vi "Merge Limelight Data.vi"   [LabVIEW 2025]
uses:
  <vilib>/Rock Robotics/Network Tables/NT Read Numeric Array.vi
  <vilib>/Rock Robotics/Network Tables/NT Read Number.vi
  Framework/Robot Global Data.vi
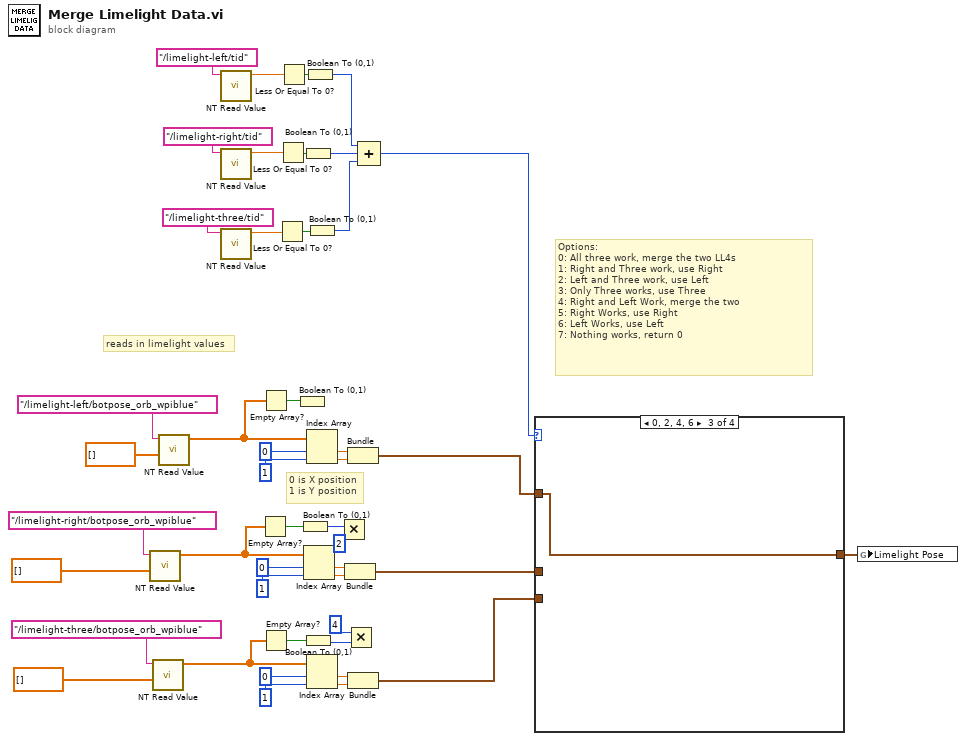
[diagram p0: block diagram]
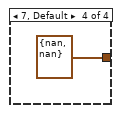
[diagram p4: hidden frame]
diagram:
  # "Options:\n0: All three work, merge the two LL4s \n1: Right and Three work, use Right\n2: Left and Three work, use Left\n3: Only Three works, use Three\n4: Right and Left Work, merge the two\n5: Right Works, use Right\n6: Left Works, use Left\n7: Nothing works, return 0"
  # "reads in limelight values"
  # "0 is X position\n1 is Y position"
  n1 = call-poly <vilib>:"NT Read Value.vi"("default value"=dbl[] [], "name"="/limelight-right/botpose_orb_wpiblue") -> ("value"=w26:dbl[])  [unwired: 7 in, 2 out]
  n2 = call-poly <vilib>:"NT Read Value.vi"("default value"=dbl[] [], "name"="/limelight-three/botpose_orb_wpiblue") -> ("value"=w25:dbl[])  [unwired: 7 in, 2 out]
  n3 = call-poly <vilib>:"NT Read Value.vi"("default value"=dbl[] [], "name"="/limelight-left/botpose_orb_wpiblue") -> ("value"=w27:dbl[])  [unwired: 7 in, 2 out]
  n4 = call-poly <vilib>:"NT Read Value.vi"("name"="/limelight-left/tid") -> ("value"=w10:dbl)  [unwired: 8 in, 2 out]
  n5 = call-poly <vilib>:"NT Read Value.vi"("name"="/limelight-right/tid") -> ("value"=w9:dbl)  [unwired: 8 in, 2 out]
  n6 = call-poly <vilib>:"NT Read Value.vi"("name"="/limelight-three/tid") -> ("value"=w8:dbl)  [unwired: 8 in, 2 out]
  n7 = Empty Array?(array=w26) -> (empty?=w23:bool)
  n8 = Empty Array?(array=w27) -> (empty?=w22:bool)
  n9 = Empty Array?(array=w25) -> (empty?=w24:bool)
  n10 = Less Or Equal To 0?(x=w8) -> (x <= 0?=w7:bool)
  n11 = Less Or Equal To 0?(x=w9) -> (x <= 0?=w6:bool)
  n12 = Less Or Equal To 0?(x=w10) -> (x <= 0?=w5:bool)
  n13 = Boolean To (0,1)(Boolean=w22) -> ()  [unwired: 1 out]
  n14 = Boolean To (0,1)(Boolean=w23) -> (0, 1=w19:i16)
  n15 = Boolean To (0,1)(Boolean=w6) -> (0, 1=w3:i16)
  n16 = Boolean To (0,1)(Boolean=w24) -> (0, 1=w21:i16)
  n17 = Index Array(array=w26, index #1=0 ("index"), index #2=1 ("index")) -> (element #1=w39:dbl, element #2=w40:dbl)
  n18 = Boolean To (0,1)(Boolean=w5) -> (0, 1=w4:i16)
  n19 = Boolean To (0,1)(Boolean=w7) -> (0, 1=w2:i16)
  n20 = Index Array(array=w27, index #1=0 ("index"), index #2=1 ("index")) -> (element #1=w44:dbl, element #2=w45:dbl)
  n21 = Index Array(array=w25, index #1=0 ("index"), index #2=1 ("index")) -> (element #1=w32:dbl, element #2=w31:dbl)
  n22 = Multiply(x=w19, y=i16 2) -> ()  [unwired: 1 out]
  n23 = Bundle("Numeric"=w39, "Numeric"=w40) -> (w16:cluster{"Numeric":dbl, "Numeric":dbl})  [unwired: 1 in]
  n24 = Multiply(x=i16 4, y=w21) -> ()  [unwired: 1 out]
  n25 = Bundle("Numeric"=w44, "Numeric"=w45) -> (w17:cluster{"Numeric":dbl, "Numeric":dbl})  [unwired: 1 in]
  n26 = Bundle("Numeric"=w32, "Numeric"=w31) -> (w15:cluster{"Numeric":dbl, "Numeric":dbl})  [unwired: 1 in]
  n27 = Compound Arithmetic op=ADD(w4, w3, w2) -> (w1:i16)
  n28 = case shown="0, 2, 4, 6" w1 {
    tunnel: w17 -> [_ _ w48 _]
    tunnel: w16 -> [w46 _ _ _]
    tunnel: w15 -> [_ w47 _ _]
    tunnel: [w46 w47 w48 cluster{"Numeric":dbl, "Numeric":dbl} {"Numeric"=nan, "Numeric"=nan}] -> w14
    frame 1, 5 {
    }
    frame 3 {
    }
    frame 0, 2, 4, 6 {
    }
    frame 7, Default {
    }
  }
  n29 = global write "Robot Global Data.vi" "Limelight Pose"(w14) -> ()
